vi "lcr tuning derivative.vi"(8 "lower limit":dbl=3.7, 9 "upper limit":dbl=3.7, 10 "lcr in":refnum<visa-resource-name>, 11 "polarimeter in":refnum<k21>) -> (1 "c8 voltage":dbl, 2 "lcr out":refnum<visa-resource-name>, 3 "polarimeter out":refnum<k21>)   [LabVIEW 2018]
uses:
  0a1fad13-b885-4eab-b2d2-ceeba4e32cbd.vi
  <vilib>/DAQmx/read.llb/DAQmx Read (Analog DBL 1Chan 1Samp).vi
  <vilib>/Analysis/baseanly.llb/Mean (DBL).vi
  <vilib>/DAQmx/miscellaneous.llb/DAQmx Fill In Error Info.vi
  <vilib>/ptbypt/NI_PtbyPt.lvlib
  <vilib>/Analysis/NI_AALBase.lvlib
panel:
  out "Derivative":dbl(graph)
  out "Average":dbl(graph)
  out "current voltage":dbl
  out "diode voltage":dbl
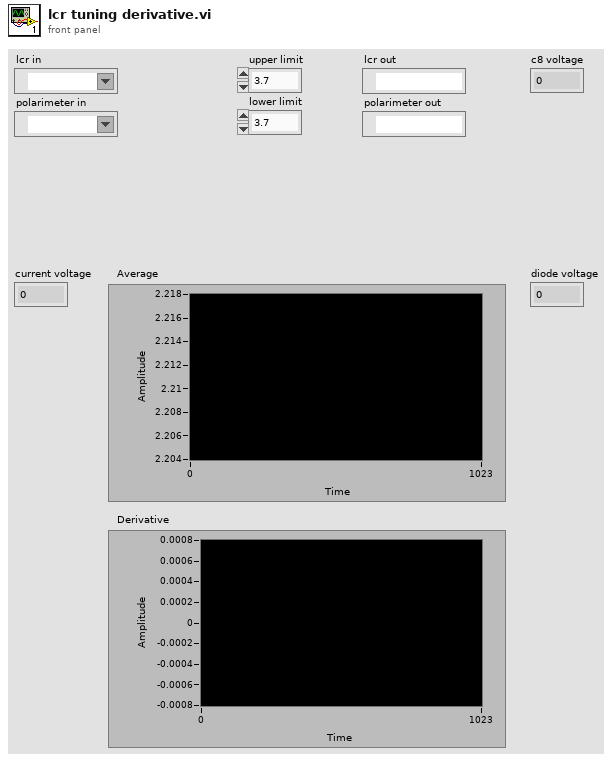
[diagram p1: front panel]
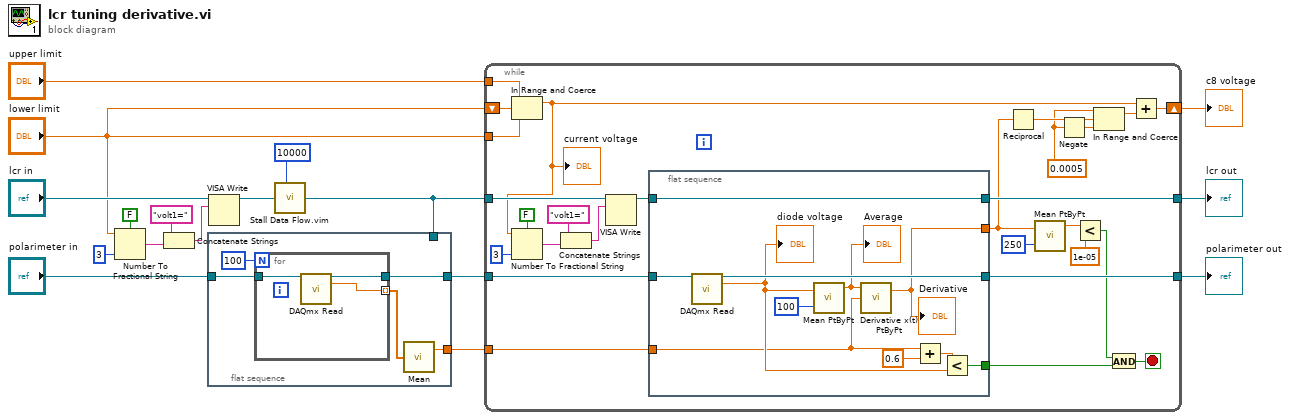
[diagram p0: block diagram]
diagram:
  n1 = Number To Fractional String(use system decimal point (T)=FALSE, number="lower limit", precision (6)=i16 3) -> (F-format string=w7:string)  [unwired: 1 in]
  n2 = Concatenate Strings("volt1=" ("string"), w7) -> (w3:string)
  n3 = flat-sequence {
    tunnel: "polarimeter in" -> [w22]
    tunnel: [w21] -> w12
    tunnel: [w18] -> w10
    tunnel: w11 -> [_]
    frame #0 {
      n4 = for {
        N: 100 -> [_]
        tunnel: [w23] -> w19 mode=indexing
        tunnel: w22 -> [w25]
        tunnel: [w24] -> w21
        n5 = call-poly <vilib>:"DAQmx Read.vi"("task/channels in"=w25) -> ("task out"=w24:refnum<k21>, "data"=w23:dbl)  [unwired: 12 in, 1 out]
      }
      n6 = call-poly <vilib>:"Mean.vi"("X"=w19) -> ("mean"=w18:dbl)  [unwired: 1 out]
    }
  }
  n7 = VISA Write(VISA resource name="lcr in", write buffer=w3) -> (VISA resource name out=w4:refnum<visa-resource-name>)  [unwired: 1 in, 2 out]
  n8 = call "Stall Data Flow.vim"("value in"=w4, "milliseconds to wait"=u32 10000) -> ("value out"=w11:refnum<visa-resource-name>)  [unwired: 1 out]
  n9 = while {
    shift-right: [w50] -> w15
    shift-left: "lower limit" -> [w49]
    tunnel: "upper limit" -> [w44]
    tunnel: "lower limit" -> [w43]
    tunnel: w12 -> [w51]
    tunnel: [w52] -> w16
    tunnel: w10 -> [w41]
    tunnel: w11 -> [w28]
    tunnel: [w42] -> w1
    stop <- w38 stop-if-true
    w46 = 0.0005 ("limit")
    n10 = In Range and Coerce(upper limit=w44, x=w49, lower limit=w43) -> (coerced(x)=w26:dbl)  [unwired: 1 out]
    "current voltage" <- w26
    n11 = Number To Fractional String(use system decimal point (T)=FALSE, number=w26, precision (6)=i16 3) -> (F-format string=w31:string)  [unwired: 1 in]
    n12 = Concatenate Strings("volt1=" ("string"), w31) -> (w27:string)
    n13 = VISA Write(VISA resource name=w28, write buffer=w27) -> (VISA resource name out=w29:refnum<visa-resource-name>)  [unwired: 1 in, 2 out]
    n14 = flat-sequence {
      tunnel: [w63] -> w52
      tunnel: w51 -> [w62]
      tunnel: w29 -> [w60]
      tunnel: [w60] -> w42
      tunnel: w41 -> [w54]
      tunnel: [w56] -> w34
      tunnel: [w55] -> w39
      frame #0 {
        n15 = call-poly <vilib>:"DAQmx Read.vi"("task/channels in"=w62) -> ("task out"=w63:refnum<k21>, "data"=w58:dbl)  [unwired: 12 in, 1 out]
        "diode voltage" <- w58
        n16 = call <vilib>:"Mean PtByPt.vi"("x"=w58, "sample length"=100) -> ("mean"=w59:dbl)  [unwired: 2 in, 1 out]
        "Average" <- w59
        n17 = call <vilib>:"Derivative x(t) PtByPt.vi"("initial condition"=w54, "x"=w59) -> ("dx/dt"=w55:dbl)  [unwired: 2 in, 1 out]
        "Derivative" <- w55
        n18 = Add(x=w54, y=0.6) -> (x+y=w57:dbl)
        n19 = Less?(x=w57, y=w58) -> (x < y?=w56:bool)
      }
    }
    n20 = Reciprocal(x=w39) -> (1/x=w48:dbl)
    n21 = call <vilib>:"Mean PtByPt.vi"("x"=w39, "sample length"=250) -> ("mean"=w36:dbl)  [unwired: 2 in, 1 out]
    n22 = Negate(x=w46) -> (-x=w45:dbl)
    n23 = Less?(x=w36, y=1e-05 ("x")) -> (x < y?=w35:bool)
    n24 = In Range and Coerce(upper limit=w46, x=w48, lower limit=w45) -> (coerced(x)=w47:dbl)  [unwired: 1 out]
    n25 = And(x=w35, y=w34) -> (x .and. y?=w38:bool)
    n26 = Add(x=w26, y=w47) -> (x+y=w50:dbl)
  }
  "polarimeter out" <- w16
  "c8 voltage" <- w15
  "lcr out" <- w1
